vi "_API_BINANCE_GET_Time.vi"(0 "BinanceAPI_.lvclass":refnum<class "BinanceAPI_.lvclass">, 11 "error in (no error)":errorcluster) -> (4 "BinanceAPI_.lvclass 2":refnum<class "BinanceAPI_.lvclass">, 6 "Time in seckond from 01.01.1970":string, 8 "Timestamp":timestamp, 15 "error out":errorcluster)   [LabVIEW 2022 SP3, in "BinanceAPI_.lvclass"]
doc: "https://binance-docs.github.io/apidocs/spot/en/#check-server-time"
uses:
  BinanceAPI_.lvclass
  BinanceAPI_.lvclass/BinanceAPI_.ctl
  <vilib>/httpClient/LabVIEWHTTPClient.lvlib
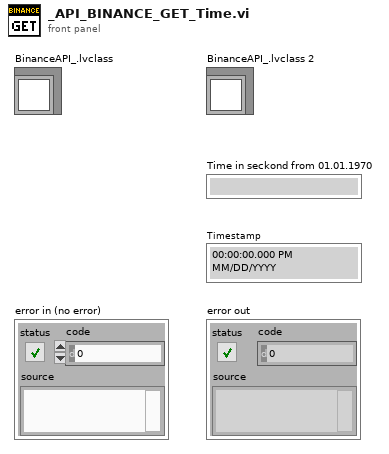
[diagram p1: front panel]
types:
  T1 = typedef "LabVIEWHTTPClient.lvlib/ClientHandle.ctl" = refnum<k1>
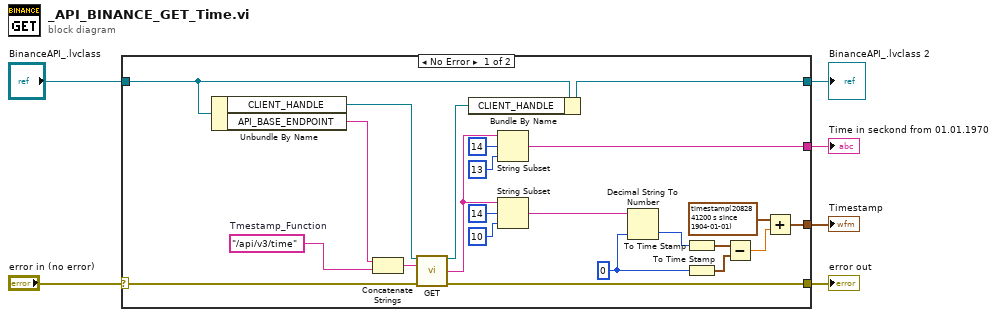
[diagram p0: block diagram]
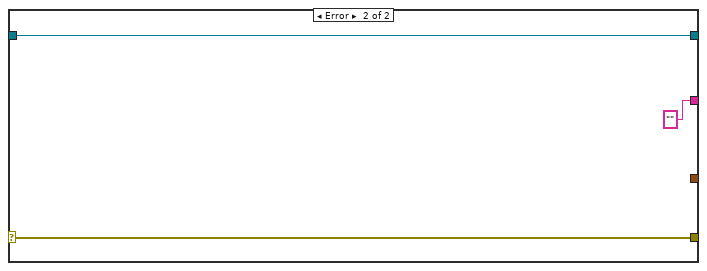
[diagram p2: hidden frame]
diagram:
  n1 = case shown="No Error" "error in (no error)" {
    selector: "error in (no error)" -> [w26 w32]
    tunnel: [w19 w32] -> w6
    tunnel: [w8 "" ("body")] -> w2
    tunnel: [w22 w30] -> w3
    tunnel: "BinanceAPI_.lvclass" -> [w23 w30]
    tunnel: [w9 _] -> w1
    frame No Error {
      w17 = i64 0 ("default (0 I32)")
      w28 = "/api/v3/time"  # Tmestamp_Function
      n2 = Unbundle By Name(w23) -> ("CLIENT_HANDLE"=w25:T1, "API_BASE_ENDPOINT"=w27:string)
      n3 = Concatenate Strings(w27, w28) -> (w29:string)
      n4 = call <vilib>:"GET.vi"("client handle"=w25, "url"=w29, "error in (no error)"=w26) -> ("client handle out"=w24:T1, "body"=w10:string, "error out"=w19:errorcluster)  [unwired: 9 in, 1 out]
      n5 = Bundle By Name(cluster=w23, "CLIENT_HANDLE"=w24) -> (w22:refnum<class "BinanceAPI_.lvclass">)
      n6 = String Subset(string=w10, offset (0)=14, length (rest)=13 ("length (rest)")) -> (substring=w8:string)
      n7 = String Subset(string=w10, offset (0)=14, length (rest)=10 ("length (rest)")) -> (substring=w7:string)
      n8 = Decimal String To Number(string=w7, default (0L)=w17) -> (number=w18:i64)  [unwired: 1 in, 1 out]
      n9 = To Time Stamp(1:w18) -> (0:w16:timestamp)
      n10 = To Time Stamp(1:w17) -> (0:w15:timestamp)
      n11 = Subtract(x=w16, y=w15) -> (x-y=w13:dbl)
      n12 = Add(x=timestamp(2082841200 s since 1904-01-01), y=w13) -> (x+y=w9:timestamp)
    }
    frame Error {
    }
  }
  "error out" <- w6
  "Time in seckond from 01.01.1970" <- w2
  "BinanceAPI_.lvclass 2" <- w3
  "Timestamp" <- w1
